vi "ip address.vi"() -> (3 "ip address":string)   [LabVIEW 2014]
panel:
  # "링크-로컬 IPv6 주소 . . . . :"
  # "서브넷 마스크"
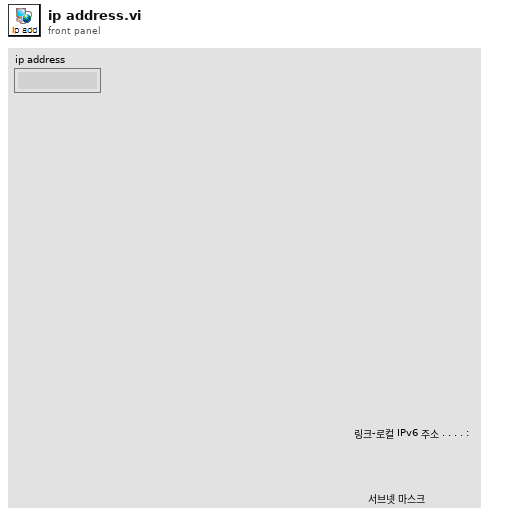
[diagram p1: front panel]
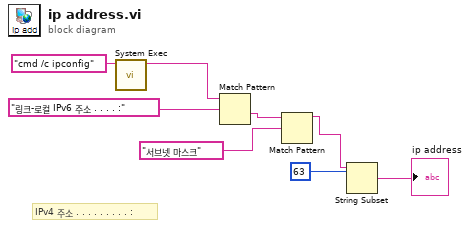
[diagram p0: block diagram]
diagram:
  # "IPv4 주소 . . . . . . . . . :"
  n1 = call <vilib>:"System Exec.vi"("command line"="cmd /c ipconfig") -> ("standard output"=w7:string)  [unwired: 7 in, 3 out]
  n2 = Match Pattern(string=w7, regular expression="링크-로컬 IPv6 주소 . . . . :" ("정규식")) -> (after substring=w5:string)  [unwired: 1 in, 3 out]
  n3 = Match Pattern(string=w5, regular expression="서브넷 마스크" ("정규식")) -> (before substring=w3:string)  [unwired: 1 in, 3 out]
  n4 = String Subset(string=w3, offset (0)=63 ("오프셋(0)")) -> (substring=→"ip address":string)  [unwired: 1 in]
